vi "Test Waveform Diogo.vi"() -> ()   [LabVIEW 2016]
uses:
  <vilib>/measure/matone.llb/Extract Single Tone Information 1 Chan.vi
  <vilib>/measure/mamon.llb/Create Continuous Mask.vi
  <vilib>/measure/mamon.llb/Limit Testing Time.vi
  <vilib>/xnet/xnet.llb/XNET Read (Signal Waveform) .vi
  <vilib>/Waveform/WDTOps.llb/WDT Append Waveforms DBL.vi
  <vilib>/Waveform/WDTOps.llb/WDT Number of Waveform Samples DBL.vi
  <vilib>/measure/matone.llb/Extract Single Tone Information N Chan.vi
  <vilib>/measure/NI_MAPro.lvlib
  <vilib>/measure/NI_MABase.lvlib
panel:
  in  "square wave duty cycle (%) down":dbl=50.0 format="%#_13g"
  in  "square wave duty cycle (%) up":dbl=50.0 format="%#_13g"
  out "detected frequency":dbl format="%.2p"
  out "detected frequencies":dbl[](array[numeric]) format="%.2p"
  out "Waveform Graph 3":dynamicdata(graph)
  in  "signal type":T1(ring)
  out "detected amplitude":dbl format="%.2p"
  in  "amplitude":dbl=1.0 format="%0.2p"
  out "test passed?":bool
  out "error out 3":errorcluster
  out "error out 2":errorcluster caption="error out"
  out "error out":errorcluster
  out "Limit 3":cluster{"x0":dbl, "dx":dbl, "Y":dbl[]} caption="Limit" {"Y" format="%.2p"; "dx" format="%.2p"; "x0" format="%.2p"}
  out "detected phase (deg)":dbl format="%.2p"
  out "Waveform Graph 2":waveform(dbl)(graph)
  out "Waveform Graph":waveform(dbl)[](graph)
  in  "stop":bool
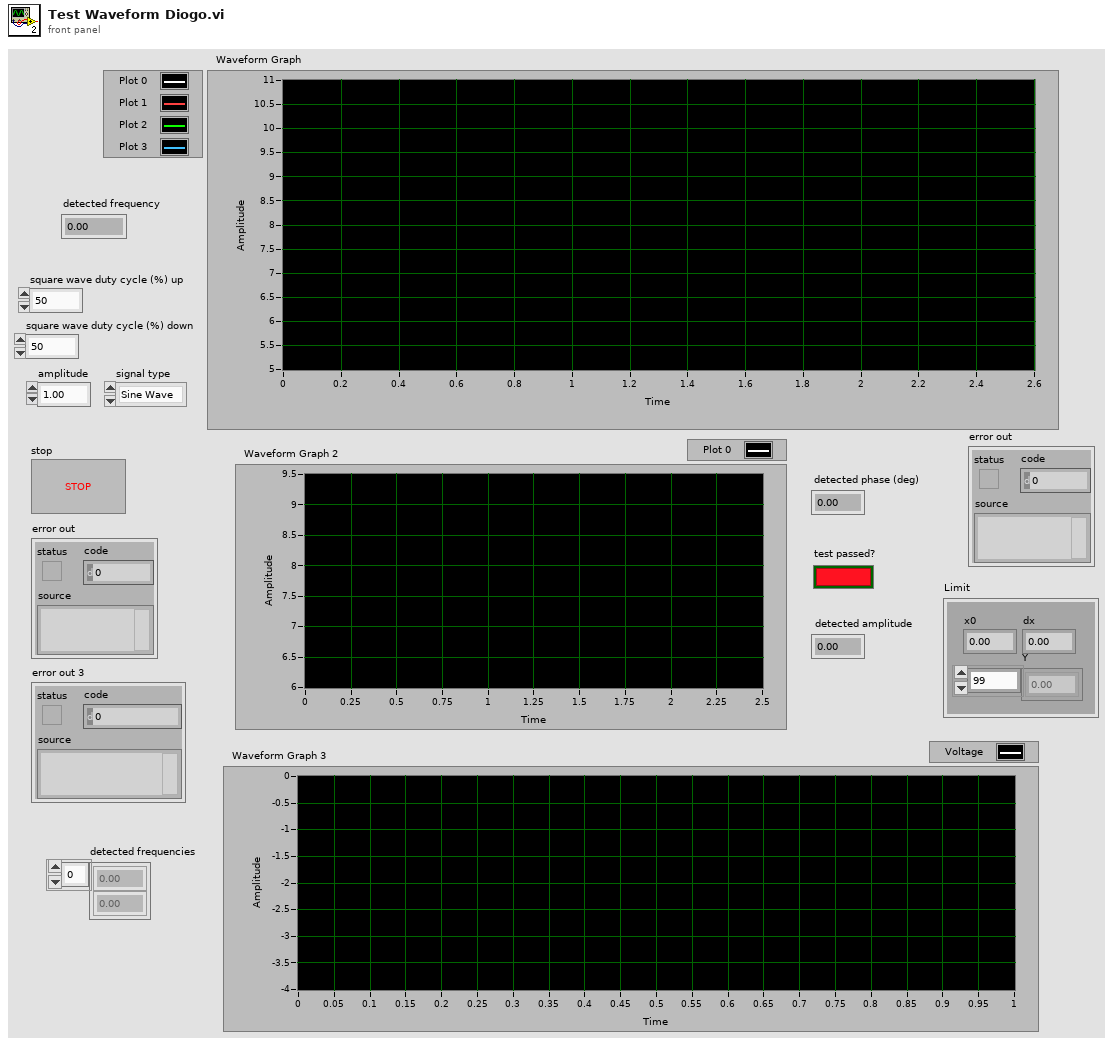
[diagram p1: front panel]
types:
  T1 = enum16{"Sine Wave", "Triangle Wave", "Square Wave", "Sawtooth Wave"}
  T2 = cluster{"pass region":i32, "include UL":bool, "include LL":bool}
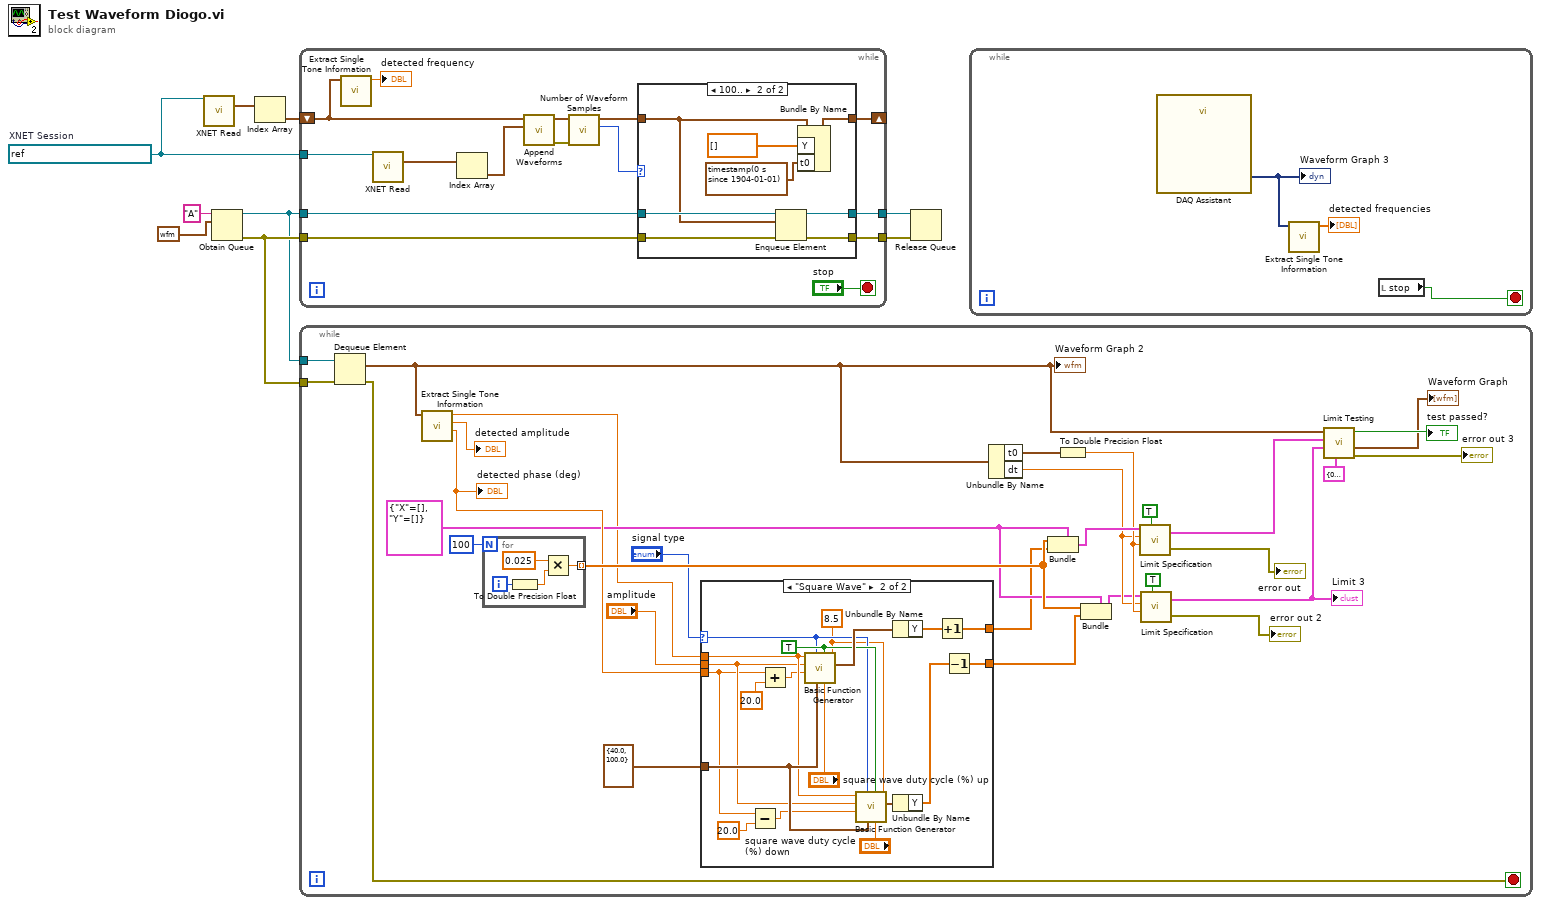
[diagram p0: block diagram]
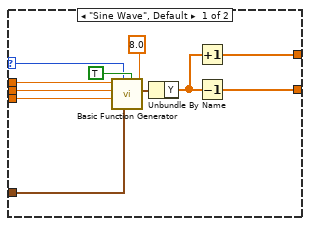
[diagram p2: hidden frame]
diagram:
  w3 = refnum<k21> "New NI-XNET Session"  # XNET Session
  n1 = call-poly <vilib>:"XNET Read.vi"("session in"=w3) -> ("data"=w4:waveform(dbl)[])  [unwired: 12 in, 2 out]
  n2 = Obtain Queue(name (unnamed)="A", element data type=waveform(dbl) {"t0"=timestamp(0 s since 1904-01-01), "dt"=1.0, "Y"=[]}) -> (queue out=w5:refnum<queue>, error out=w6:errorcluster)  [unwired: 3 in, 1 out]
  n3 = Index Array(array=w4) -> (element=w2:waveform(dbl))  [unwired: 1 in]
  n4 = while {
    tunnel: w3 -> [w24]
    tunnel: w5 -> [w22]
    tunnel: [w21] -> w9
    tunnel: [w20] -> w1
    tunnel: w6 -> [w19]
    shift-right: [w12] -> _
    shift-left: w2 -> [w11]
    stop <- "stop" stop-if-true
    n5 = call-poly <vilib>:"Extract Single Tone Information.vi"("time signal in"=w11) -> ("detected frequency"=→"detected frequency":dbl)  [unwired: 5 in, 5 out]
    n6 = call-poly <vilib>:"XNET Read.vi"("session in"=w24) -> ("data"=w18:waveform(dbl)[])  [unwired: 12 in, 2 out]
    n7 = Index Array(array=w18) -> (element=w17:waveform(dbl))  [unwired: 1 in]
    n8 = call-poly <vilib>:"Append Waveforms.vi"("waveform B"=w17, "waveform A"=w11) -> ("error out"=w16:errorcluster, "waveform out"=w15:waveform(dbl))  [unwired: 8 in]
    n9 = call-poly <vilib>:"Number of Waveform Samples.vi"("error in (no error)"=w16, "waveform in"=w15) -> ("number of samples"=w14:i32, "waveform out"=w13:waveform(dbl))  [unwired: 7 in, 1 out]
    n10 = case shown="100.." w14 {
      tunnel: w22 -> [w26 w35]
      tunnel: [w26 w34] -> w21
      tunnel: [w25 w33] -> w20
      tunnel: w19 -> [w25 w32]
      tunnel: w13 -> [w27 w31]
      tunnel: [w27 w30] -> w12
      frame 0, Default {
      }
      frame 100.. {
        n11 = Enqueue Element(queue=w35, element=w31, error in (no error)=w32) -> (queue out=w34:refnum<queue>, error out=w33:errorcluster)  [unwired: 1 in, 1 out]
        n12 = Bundle By Name(cluster=w31, "Y"=dbl[] [], "t0"=timestamp(0 s since 1904-01-01)) -> (w30:waveform(dbl))
      }
    }
  }
  n13 = while {
    tunnel: w5 -> [w65]
    tunnel: w6 -> [w64]
    stop <- w63 stop-if-true
    w45 = cluster{"X":dbl[], "Y":dbl[]} {"X"=[], "Y"=[]} ("Specification Cluster")
    n14 = Dequeue Element(queue=w65, error in (no error)=w64) -> (element=w46:waveform(dbl), error out=w63:errorcluster)  [unwired: 1 in, 2 out]
    "Waveform Graph 2" <- w46
    n15 = call-poly <vilib>:"Extract Single Tone Information.vi"("time signal in"=w46) -> ("detected phase (deg)"=w57:dbl, "detected amplitude"=→"detected amplitude":dbl, "detected frequency"=w41:dbl)  [unwired: 5 in, 3 out]
    "detected phase (deg)" <- w57
    n16 = for {
      N: 100 -> [_]
      tunnel: [w99] -> w59 mode=indexing
      i -> [w97]
      n17 = To Double Precision Float(number=w97) -> (double precision float=w96:dbl)
      n18 = Multiply(x=0.025 ("y"), y=w96) -> (x*y=w99:dbl)
    }
    n19 = case shown="\"Square Wave\"" "signal type" {
      selector: "signal type" -> [w70 w88]
      tunnel: cluster{"Fs":dbl, "#s":dbl} {"Fs"=40.0, "#s"=100.0} ("sampling info") -> [w76 w90]
      tunnel: w57 -> [w74 w78]
      tunnel: "amplitude" -> [w72 w85]
      tunnel: w41 -> [w71 w86]
      tunnel: [w68 w83] -> w37
      tunnel: [w66 w82] -> w36
      frame "Sine Wave", Default {
        n20 = call <vilib>:"Basic Function Generator.vi"("offset"=8.0, "reset signal"=TRUE, "sampling info"=w76, "signal type"=w70, "phase"=w74, "amplitude"=w72, "frequency"=w71) -> ("signal out"=w69:waveform(dbl))  [unwired: 2 in, 2 out]
        n21 = Unbundle By Name(w69) -> ("Y"=w67:dbl[])
        n22 = Increment(x=w67) -> (x+1=w68:dbl[])
        n23 = Decrement(x=w67) -> (x-1=w66:dbl[])
      }
      frame "Square Wave" {
        w89 = TRUE ("reset signal")
        w87 = 8.5 ("offset")
        n24 = Subtract(x=w78, y=20.0) -> (x-y=w79:dbl)
        n25 = Add(x=w78, y=20.0) -> (x+y=w81:dbl)
        n26 = call <vilib>:"Basic Function Generator.vi"("offset"=w87, "square wave duty cycle (%)"="square wave duty cycle (%) up", "reset signal"=w89, "sampling info"=w90, "signal type"=w88, "phase"=w81, "amplitude"=w85, "frequency"=w86) -> ("signal out"=w94:waveform(dbl))  [unwired: 1 in, 2 out]
        n27 = call <vilib>:"Basic Function Generator.vi"("offset"=w87, "square wave duty cycle (%)"="square wave duty cycle (%) down", "reset signal"=w89, "sampling info"=w90, "signal type"=w88, "phase"=w79, "amplitude"=w85, "frequency"=w86) -> ("signal out"=w93:waveform(dbl))  [unwired: 1 in, 2 out]
        n28 = Unbundle By Name(w94) -> ("Y"=w92:dbl[])
        n29 = Unbundle By Name(w93) -> ("Y"=w91:dbl[])
        n30 = Increment(x=w92) -> (x+1=w83:dbl[])
        n31 = Decrement(x=w91) -> (x-1=w82:dbl[])
      }
    }
    n32 = Unbundle By Name(w46) -> ("t0"=w54:timestamp, "dt"=w52:dbl)
    n33 = Bundle(cluster=w45, "X"=w59, "Y"=w37) -> (w62:cluster{"X":dbl[], "Y":dbl[]})
    n34 = To Double Precision Float(number=w54) -> (double precision float=w53:dbl)
    n35 = Bundle(cluster=w45, "X"=w59, "Y"=w36) -> (w47:cluster{"X":dbl[], "Y":dbl[]})
    n36 = call-poly <vilib>:"Limit Specification.vi"("Specification Cluster"=w62, "dx"=w52, "x0"=w53, "Reset"=TRUE) -> ("Limit"=w56:cluster{"x0":dbl, "dx":dbl, "Y":dbl[]}, "error out"=→"error out":errorcluster)  [unwired: 1 in]
    n37 = call-poly <vilib>:"Limit Specification.vi"("Specification Cluster"=w47, "dx"=w52, "x0"=w53, "Reset"=TRUE) -> ("Limit"=w48:cluster{"x0":dbl, "dx":dbl, "Y":dbl[]}, "error out"=→"error out 2":errorcluster)  [unwired: 1 in]
    "Limit 3" <- w48
    n38 = call-poly <vilib>:"Limit Testing.vi"("limit test config"=T2 {"pass region"=0, "include UL"=TRUE, "include LL"=TRUE}, "lower limit"=w48, "upper limit"=w56, "signal in"=w46) -> ("error out"=→"error out 3":errorcluster, "output values"=→"Waveform Graph":waveform(dbl)[], "test passed?"=→"test passed?":bool)  [unwired: 2 in, 3 out]
  }
  n39 = Release Queue(queue=w9, error in (no error)=w1) -> ()  [unwired: 1 in, 3 out]
  n40 = while {
    stop <- w102 stop-if-true
    n41 = call "DAQ Assistant"() -> ("data"=w101:dynamicdata)  [unwired: 16 in, 3 out]
    "Waveform Graph 3" <- w101
    n42 = call-poly <vilib>:"Extract Single Tone Information.vi"("time signals in"=w101) -> ("detected frequencies"=→"detected frequencies":dbl[])  [unwired: 5 in, 5 out]
    n43 = local read "stop"() -> (w102:bool)
  }
